vi "Test to String on Non String Array.vi"() -> ()   [LabVIEW 2020, in "Basic.Mechanics.Tests.lvclass"]
uses:
  Basic.Mechanics.Tests.lvclass
  9135ef9e-d12d-4b43-94c9-f225a9f79933.vi
  9135ef9e-d12d-4b43-94c9-f225a9f79933.vi/5b84c07b-8b36-46ce-878d-0b3558e12aa4.vi
  9135ef9e-d12d-4b43-94c9-f225a9f79933.vi/5b84c07b-8b36-46ce-878d-0b3558e12aa4.vi/b30c0498-5c87-4a37-a7a8-8ea35c3fd313.vi
  <vilib>/addons/_JKI Toolkits/Caraya/classes/Assert/Assert Equal Value and Type_Variant.vi
  Basic.Mechanics.Tests.lvclass/Basic.Mechanics.Tests.ctl
  <vilib>/addons/_JKI Toolkits/Caraya/classes/Test/Test.lvclass
  <vilib>/addons/_JKI Toolkits/Caraya/classes/Assert/Assert.lvclass
panel:
  out "log string":string
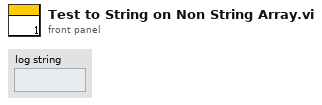
[diagram p1: front panel]
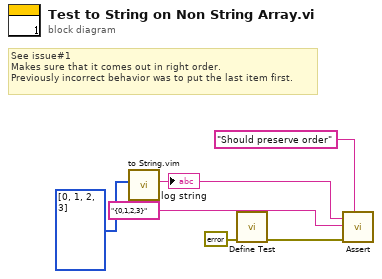
[diagram p0: block diagram]
diagram:
  # "See issue#1\nMakes sure that it comes out in right order.\nPreviously incorrect behavior was to put the last item first."
  n1 = call "to String.vim"("Anything"=i32[] [0, 1, 2, 3]) -> ("log string"=w1:string)  [unwired: 10 in]
  "log string" <- w1
  n2 = call <vilib>:"Define Test.vi"("error in (no error)"=errorcluster {"status"=FALSE, "code"=0, "source"=""}) -> ("error out"=w6:errorcluster)  [unwired: 9 in, 1 out]
  n3 = call-poly <vilib>:"Assert.vi"("Label"="Should preserve order" ("Label (VI Title)"), "error in (no error)"=w6, "Y"="{0,1,2,3}" ("log string"), "X"=w1) -> ()  [unwired: 6 in, 2 out]
